vi "Add Error Status Channels.vi"(8 "error in":errorcluster, 11 "status section ref":T1 format="%.0x") -> (0 "error out":errorcluster, 3 "status section ref out":T1 format="%.0x")   [LabVIEW 2020, in "Ballard ARINC 429 Scripting.lvlib"]
uses:
  Ballard ARINC 429 Scripting.lvlib
  <vilib>/NI VeriStand/Custom Device API/Custom Device Item Ref.ctl
  <vilib>/NI VeriStand/Custom Device API/Custom Device Channel.ctl
  <vilib>/NI VeriStand/Custom Device API/Custom Device Channel Type.ctl
  Constants.vi
  <vilib>/NI VeriStand/Custom Device API/Custom Device API.lvlib
  <vilib>/NI VeriStand/Custom Device Offline API/Custom Device Offline API.lvlib
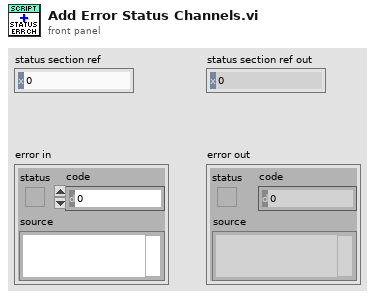
[diagram p1: front panel]
types:
  T1 = typedef "Custom Device API.lvlib/Custom Device Item Ref.ctl" = u64
  T2 = typedef "Custom Device API.lvlib/Custom Device Channel.ctl" = cluster{"Type":T3, "Units":string, "Default Value":dbl, "Faultable":bool, "Scalable":bool}
  T3 = typedef "Custom Device API.lvlib/Custom Device Channel Type.ctl" = enum16{"Input", "Output"}
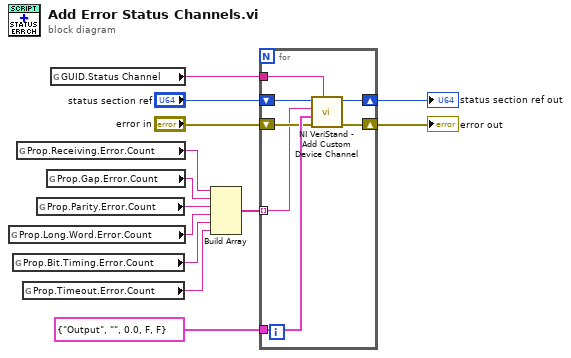
[diagram p0: block diagram]
diagram:
  n1 = global read "Constants.vi" "Prop.Long.Word.Error.Count"() -> (w3:string)
  n2 = global read "Constants.vi" "Prop.Bit.Timing.Error.Count"() -> (w4:string)
  n3 = global read "Constants.vi" "Prop.Receiving.Error.Count"() -> (w7:string)
  n4 = global read "Constants.vi" "Prop.Timeout.Error.Count"() -> (w2:string)
  n5 = global read "Constants.vi" "Prop.Parity.Error.Count"() -> (w5:string)
  n6 = global read "Constants.vi" "Prop.Gap.Error.Count"() -> (w6:string)
  n7 = global read "Constants.vi" "GUID.Status Channel"() -> (w9:string)
  n8 = Build Array(w7, w6, w5, w3, w4, w2) -> (w1:string[])
  n9 = for {
    tunnel: w9 -> [w19]
    tunnel: T2 {"Type"=enum."Output", "Units"="", "Default Value"=0.0, "Faultable"=FALSE, "Scalable"=FALSE} ("Channel") -> [w18]
    shift-right: [w15] -> w11
    shift-left: "status section ref" -> [w20]
    shift-right: [w16] -> w12
    shift-left: "error in" -> [w17]
    tunnel: w1 -> [w14] mode=indexing
    n10 = call <vilib>:"NI VeriStand - Add Custom Device Channel.vi"("GUID (Default Channel)"=w19, "error in (no error)"=w17, "Channel"=w18, "Channel Name"=w14, "Parent Ref in"=w20) -> ("error out"=w16:errorcluster, "Parent Ref out"=w15:T1)  [unwired: 3 in, 2 out]
  }
  "error out" <- w12
  "status section ref out" <- w11
